vi "Configure Trigger.vi"(4 "Trigger Delay (0 sec)":dbl, 6 "Trigger Source (0: Immediate)":u16(ring) items=["Immediate", "Trigger Link"], 8 "error in (no error)":errorcluster, 9 "Timer Setting (0.01)":dbl=0.01, 10 "Arming Source  (0: Immediate)":u16(ring) items=["Immediate", "Software Bus", "Timer", "Manual", "Trigger Link", "Rising SOT Pulse", "Falling SOT Pulse", "Rising or Falling SOT Pulse"], 11 "VISA resource name":refnum<visa-resource-name>) -> (0 "error out":errorcluster, 3 "VISA resource name out":refnum<visa-resource-name>)   [LabVIEW 2021, in "Keithley 24XX.lvlib"]
doc: "Configures the trigger settings on the instrument.\n\n<B>Note</B> Use this VI only with other low-level VIs. The high-level VIs automatically incorporate this functionality. This VI does not check the instrument status. If you want to check the instrument status, call the Error Query VI at the conclusion of the sequence."
uses:
  <instrlib>/Keithley 24XX/Keithley 24XX.lvlib
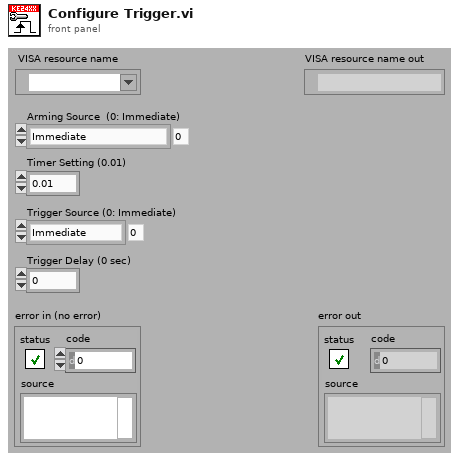
[diagram p1: front panel]
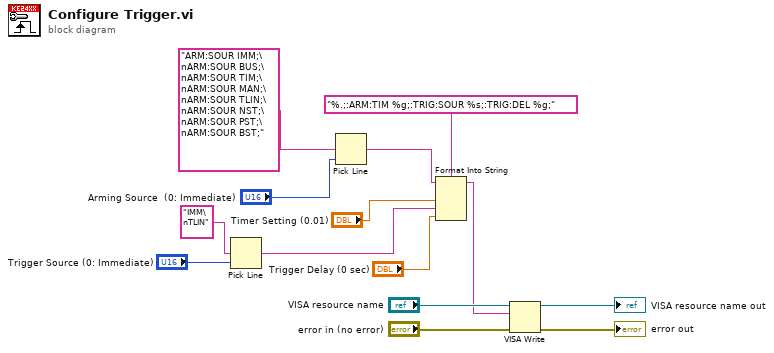
[diagram p0: block diagram]
diagram:
  n1 = Pick Line(multi-line string="IMM\nTLIN", line index="Trigger Source (0: Immediate)") -> (output string=w4:string)  [unwired: 1 in]
  n2 = Pick Line(multi-line string="ARM:SOUR IMM;\nARM:SOUR BUS;\nARM:SOUR TIM;\nARM:SOUR MAN;\nARM:SOUR TLIN;\nARM:SOUR NST;\nARM:SOUR PST;\nARM:SOUR BST;", line index="Arming Source  (0: Immediate)") -> (output string=w10:string)  [unwired: 1 in]
  n3 = Format Into String(format string="%.;:ARM:TIM %g;:TRIG:SOUR %s;:TRIG:DEL %g;", initial string=w10, "Timer Setting (0.01)", w4, "Trigger Delay (0 sec)") -> (resulting string=w7:string)  [unwired: 1 in, 1 out]
  n4 = VISA Write(VISA resource name="VISA resource name", write buffer=w7, error in (no error)="error in (no error)") -> (VISA resource name out=→"VISA resource name out":refnum<visa-resource-name>, error out=→"error out":errorcluster)  [unwired: 1 out]
